vi "05-数组和簇.vi"() -> ()   [LabVIEW 2025]
panel:
  out "Boolean":bool
  in  "布尔":bool
  out "元素":dbl
  in  "Cluster":cluster{"数值":dbl, "布尔":bool}
  out "数组大小":dbl[](array[numeric])
  out "Array 2":bool[](array[boolean])
  in  "Array":dbl[][](array[numeric])
  # "行索引"
  # "列索引"
  # "该按钮可以控制后面的小灯"
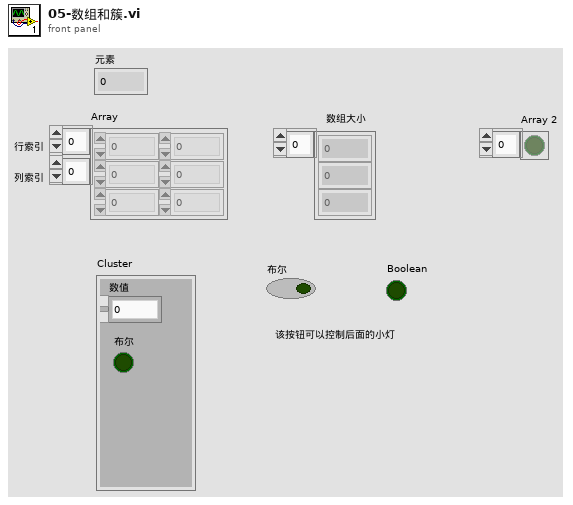
[diagram p1: front panel]
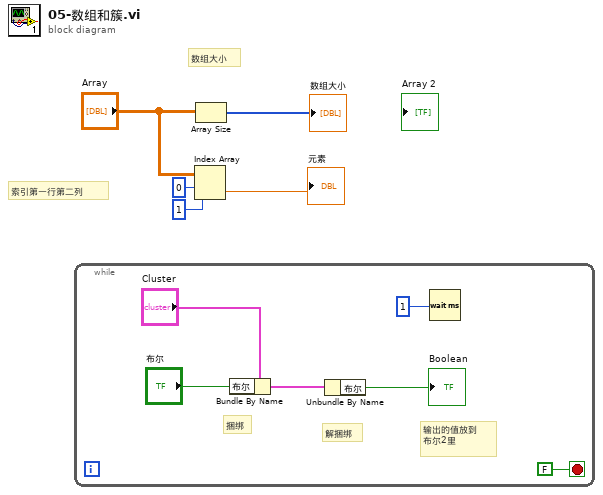
[diagram p0: block diagram]
diagram:
  # "索引第一行第二列"
  # "数组大小"
  n1 = while {
    stop <- FALSE stop-if-true
    # "输出的值放到\n布尔2里"
    # "解捆绑"
    # "捆绑"
    n2 = Bundle By Name(cluster="Cluster", "布尔"="布尔") -> (w9:cluster{"数值":dbl, "布尔":bool})
    n3 = Unbundle By Name(w9) -> ("布尔"=→"Boolean":bool)
    n4 = Wait (ms)(milliseconds to wait=u32 1 ("millisecond timer value")) -> ()  [unwired: 1 out]
  }
  n5 = Index Array(array="Array", index (row)=0, index (col)=1 ("disabled index (col)")) -> (element=→"元素":dbl)
  n6 = Array Size(array="Array") -> (size(s)=→"数组大小":i32[])
